vi "Host - Get Slaves.vi"(8 "error in (no error)":errorcluster, 11 "Master Ref in":refnum<k21>) -> (0 "error out":errorcluster, 2 "Slaves":T1[](array[typedef]), 3 "Master Ref out":refnum<k21>)   [LabVIEW 2020, in "SEECD System Explorer.lvlib"]
uses:
  SEECD System Explorer.lvlib
  Type Defs/Host - Slave.ctl
  Type Defs/Host - Module.ctl
  Type Defs/IOV Container Contents.ctl
  <resource>/objmgr/IndComECAT.rc
  1018482e-9101-47f5-a04f-1eafd3339973.vi
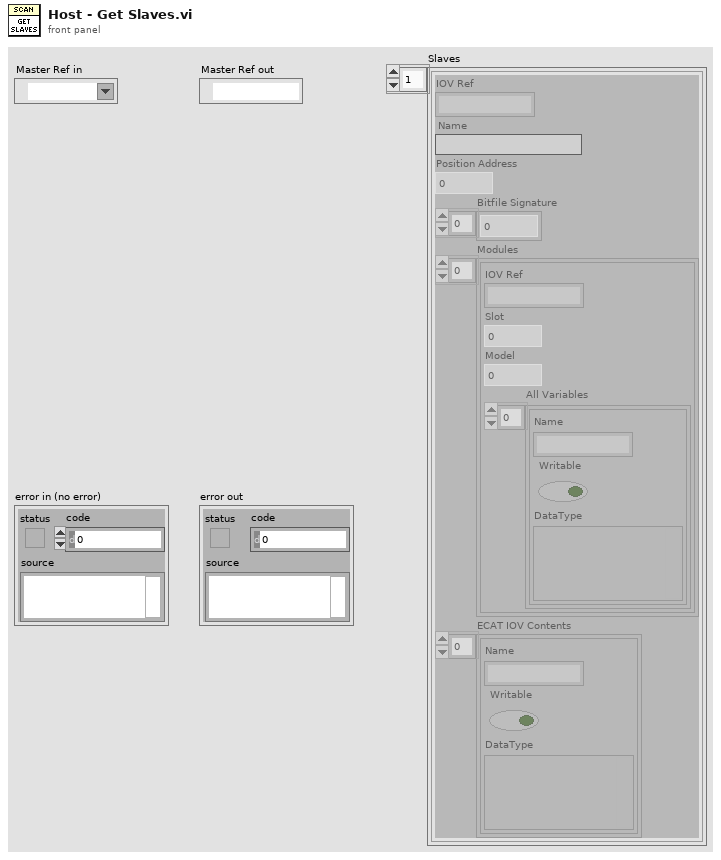
[diagram p1: front panel]
types:
  T1 = typedef "SEECD System Explorer.lvlib/Host - Slave.ctl" = cluster{"IOV Ref":string, "Name":string, "Position Address":u16, "Bitfile Signature":u8[], "Modules":T2[], "ECAT IOV Contents":T3[]}
  T2 = typedef "SEECD System Explorer.lvlib/Host - Module.ctl" = cluster{"IOV Ref":string, "Slot":u32, "Model":u32, "All Variables":T3[]}
  T3 = typedef "SEECD System Explorer.lvlib/IOV Container Contents.ctl" = cluster{"Name":string, "Writable":bool, "DataType":variant}
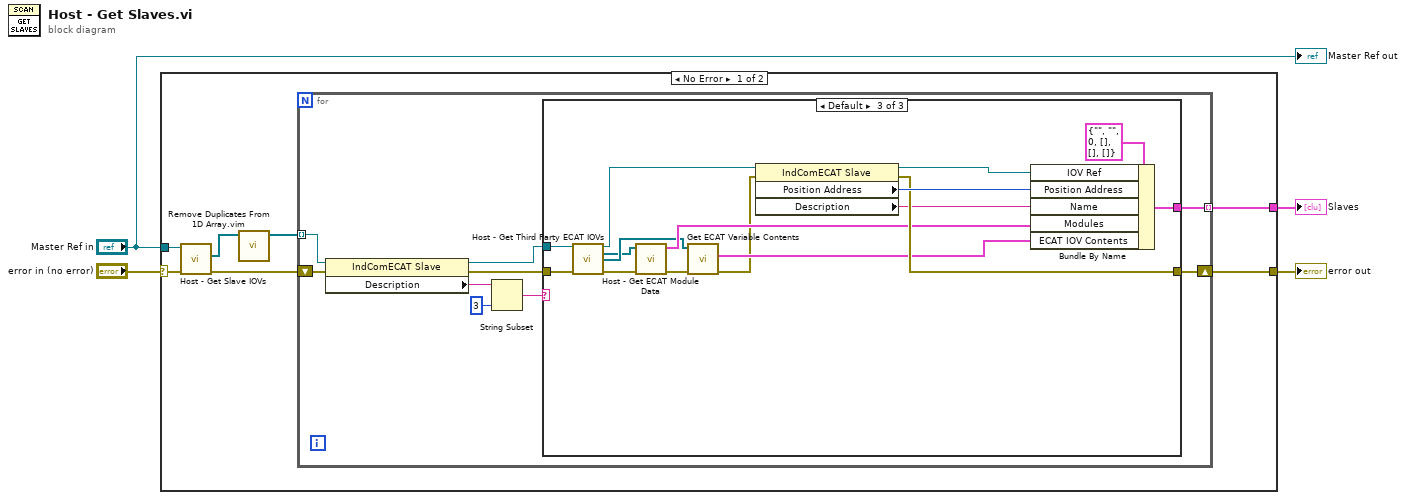
[diagram p0: block diagram]
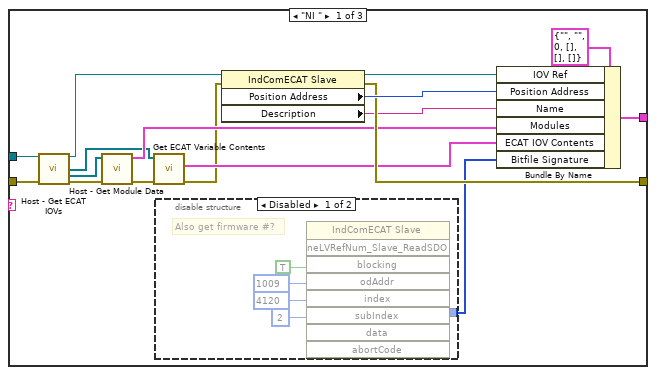
[diagram p2: hidden frame]
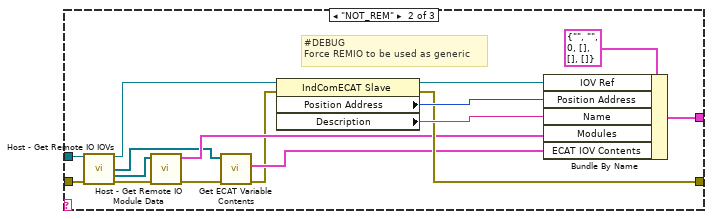
[diagram p4: hidden frame]
diagram:
  n1 = case shown="No Error" "error in (no error)" {
    selector: "error in (no error)" -> [w7 w75]
    tunnel: [w11 _] -> w4
    tunnel: [w10 w75] -> w3
    tunnel: "Master Ref in" -> [w9 _]
    frame No Error {
      n2 = call "Host - Get Slave IOVs.vi"("error in (no error)"=w7, "ECAT Master in"=w9) -> ("error IO"=w8:errorcluster, "All Slaves"=w6:refnum<k21>[])  [unwired: 7 in, 1 out]
      n3 = call "Remove Duplicates From 1D Array.vim"("array"=w6) -> ("array with duplicates removed"=w5:refnum<k21>[])  [unwired: 10 in]
      n4 = for {
        tunnel: w5 -> [w16] mode=indexing
        tunnel: [w19] -> w11 mode=indexing
        shift-right: [w18] -> w10
        shift-left: w8 -> [w20]
        n5 = property class="IndComECAT Slave"(reference=w16, error in=w20) -> (reference out=w15:refnum<k21>, error out=w17:errorcluster, "Description"=w14:string)
        n6 = String Subset(string=w14, length (rest)=3 ("length (rest)")) -> (substring=w12:string)  [unwired: 1 in]
        n7 = case shown="Default" w12 {
          tunnel: [w33 w53 w70] -> w19
          tunnel: [w32 w54 w69] -> w18
          tunnel: w17 -> [w29 w52 w66]
          tunnel: w15 -> [w28 w51 w65]
          frame "NI " {
            n8 = call "Host - Get ECAT IOVs.vi"("ECAT Slave in"=w28, "error in (no error)"=w29) -> ("ECAT Slave out"=w37:refnum<k21>, "ECAT Variablenobjekt"=w26:refnum<k21>[], "All Mods"=w21:refnum<k21>[], "error IO"=w22:errorcluster)  [unwired: 9 in, 1 out]
            n9 = call "Host - Get Module Data.vi"("error in (no error)"=w22, "Mod IOVs"=w21) -> ("error out"=w27:errorcluster, "Modules"=w30:T2[])  [unwired: 8 in]
            n10 = call "Get ECAT Variable Contents.vi"("error in (no error)"=w27, "ECAT Variablenobjekt in"=w26) -> ("error out"=w23:errorcluster, "All Variables Contents"=w24:T3[])  [unwired: 7 in, 1 out]
            n11 = disable-structure shown="Disabled" {
              disable-tunnel: [w38 _] -> w25
              frame Disabled {
                # "Also get firmware #?"
                n12 = invoke class="IndComECAT Slave" method="neLVRefNum_Slave_ReadSDO"("blocking"=TRUE, "odAddr"=u16 1009, "index"=u16 4120, "subIndex"=u8 2) -> ("data"=w38:u8[])  [unwired: 5 in, 8 out]
              }
              frame Enabled {
              }
            }
            n13 = property class="IndComECAT Slave"(reference=w37, error in=w23) -> (reference out=w35:refnum<k21>, error out=w32:errorcluster, "Position Address"=w34:u16, "Description"=w31:string)
            n14 = Bundle By Name(cluster=T1 {"IOV Ref"="", "Name"="", "Position Address"=0, "Bitfile Signature"=[], "Modules"=[], "ECAT IOV Contents"=[]} ("Slave"), "IOV Ref"=w35, "Position Address"=w34, "Name"=w31, "Modules"=w30, "ECAT IOV Contents"=w24, "Bitfile Signature"=w25) -> (w33:T1)
          }
          frame "NOT_REM" {
            # "#DEBUG\nForce REMIO to be used as generic"
            n15 = call "Host - Get Remote IO IOVs.vi"("ECAT Slave in"=w51, "error in (no error)"=w52) -> ("ECAT Slave out"=w50:refnum<k21>, "ECAT Variablenobjekt"=w45:refnum<k21>[], "All Remote IO Mods"=w47:refnum<k21>[], "error IO"=w49:errorcluster)  [unwired: 9 in, 1 out]
            n16 = call "Host - Get Remote IO Module Data.vi"("error in (no error)"=w49, "Remote IO Mod IOVs"=w47) -> ("error out"=w46:errorcluster, "Modules"=w48:T2[])  [unwired: 8 in]
            n17 = call "Get ECAT Variable Contents.vi"("error in (no error)"=w46, "ECAT Variablenobjekt in"=w45) -> ("error out"=w43:errorcluster, "All Variables Contents"=w44:T3[])  [unwired: 7 in, 1 out]
            n18 = property class="IndComECAT Slave"(reference=w50, error in=w43) -> (reference out=w56:refnum<k21>, error out=w54:errorcluster, "Position Address"=w57:u16, "Description"=w58:string)
            n19 = Bundle By Name(cluster=T1 {"IOV Ref"="", "Name"="", "Position Address"=0, "Bitfile Signature"=[], "Modules"=[], "ECAT IOV Contents"=[]} ("Slave"), "IOV Ref"=w56, "Position Address"=w57, "Name"=w58, "Modules"=w48, "ECAT IOV Contents"=w44) -> (w53:T1)
          }
          frame Default {
            n20 = call "Host - Get Third Party ECAT IOVs.vi"("ECAT Slave in"=w65, "error in (no error)"=w66) -> ("ECAT Slave out"=w74:refnum<k21>, "ECAT Modules"=w59:refnum<k21>[], "ECAT Variablenobjekt"=w63:refnum<k21>[], "error IO"=w60:errorcluster)  [unwired: 10 in]
            n21 = call "Host - Get ECAT Module Data.vi"("error in (no error)"=w60, "ECAT Modules"=w59) -> ("error out"=w64:errorcluster, "Modules"=w67:T2[])  [unwired: 8 in]
            n22 = call "Get ECAT Variable Contents.vi"("error in (no error)"=w64, "ECAT Variablenobjekt in"=w63) -> ("error out"=w61:errorcluster, "All Variables Contents"=w62:T3[])  [unwired: 7 in, 1 out]
            n23 = property class="IndComECAT Slave"(reference=w74, error in=w61) -> (reference out=w72:refnum<k21>, error out=w69:errorcluster, "Position Address"=w71:u16, "Description"=w68:string)
            n24 = Bundle By Name(cluster=T1 {"IOV Ref"="", "Name"="", "Position Address"=0, "Bitfile Signature"=[], "Modules"=[], "ECAT IOV Contents"=[]} ("Slave"), "IOV Ref"=w72, "Position Address"=w71, "Name"=w68, "Modules"=w67, "ECAT IOV Contents"=w62) -> (w70:T1)
          }
        }
      }
    }
    frame Error {
    }
  }
  "Slaves" <- w4
  "error out" <- w3
  "Master Ref out" <- "Master Ref in"
